vi "Impedance_Static_Temp.vi"() -> ()   [LabVIEW 2018]
uses:
  <vilib>/Utility/file.llb/Write Delimited Spreadsheet (DBL).vi
  <instrlib>/Agilent 4194/Agilent 4194.lvlib
panel:
  in  "Sample Thickness (micron)":dbl
  in  "Electrode Diameter (mm)":dbl
  out "error out":errorcluster
  out "Imaginary Permittivity":T1(graph)
  out "Real Permittivity":T1(graph)
  in  "STOP A":bool
  in  "Start Impedance Collection":bool
  in  "Gain-Phase (0:Tch/Rch [dB] - Theta)":u32(ring) items=["Tch/Rch [dB] - Theta", "Tch/Rch - theta", "Tch/Rch [dB] - tau", "Tch-Rch [V]", "Tch-Rch [dBm]", "Tch-Rch [dBV]"]
  in  "Sweep Type (F:Linear)":bool
  in  "Stop/Span (10,00E-3)":dbl=15000000.0 format="%^.1e"
  in  "Start/Center (10,00E-3)":dbl=100.0 min=-40.0 max=40000000.0 format="%^.3e"
  in  "Display Mode (0:X - A&B)":u32(ring) items=["X - A&B", "A - B", "Table"]
  in  "Number Of Points (100)":i32=400 min=2 max=401
  in  "Averaging Number (8:256)":u32(ring) items=["1", "2", "4", "8", "16", "32", "64", "128", "256"]
  in  "Integration Time (0:Short)":u32(ring) items=["Short", "Medium", "Long"]
  in  "Impedance (0:| Z | - Theta )":u32(ring) items=["| Z | -Ttheta ", "R - X", "Ls-Rs", "Ls-Q", "Cs-Rs", "Cs-Q", "Cs-D", "|Y|-Theta", "G-B", "Lp-G", "Lp-Q", "Cp-G", "Cp-Q", "Cp-D", "|Z|-Ls", "|Z|-Cs", "|Z|-Lp", "|Z|-Cp", "Lp-Rp", "Cp-Rp"]
  in  "Measurement Type (0:Impedance)":u32(ring) items=["Impedance ", "Gain - Phase", "Impedance With Probe"]
  in  "File Base Name":string
  in  "VISA resource name 2":refnum<visa-resource-name>="GPIB0::17::INSTR"
  out "Capacitance":T1(graph)
  out "Dissipation":T1(graph)
  in  "Force Quit":bool
  out "Status":string
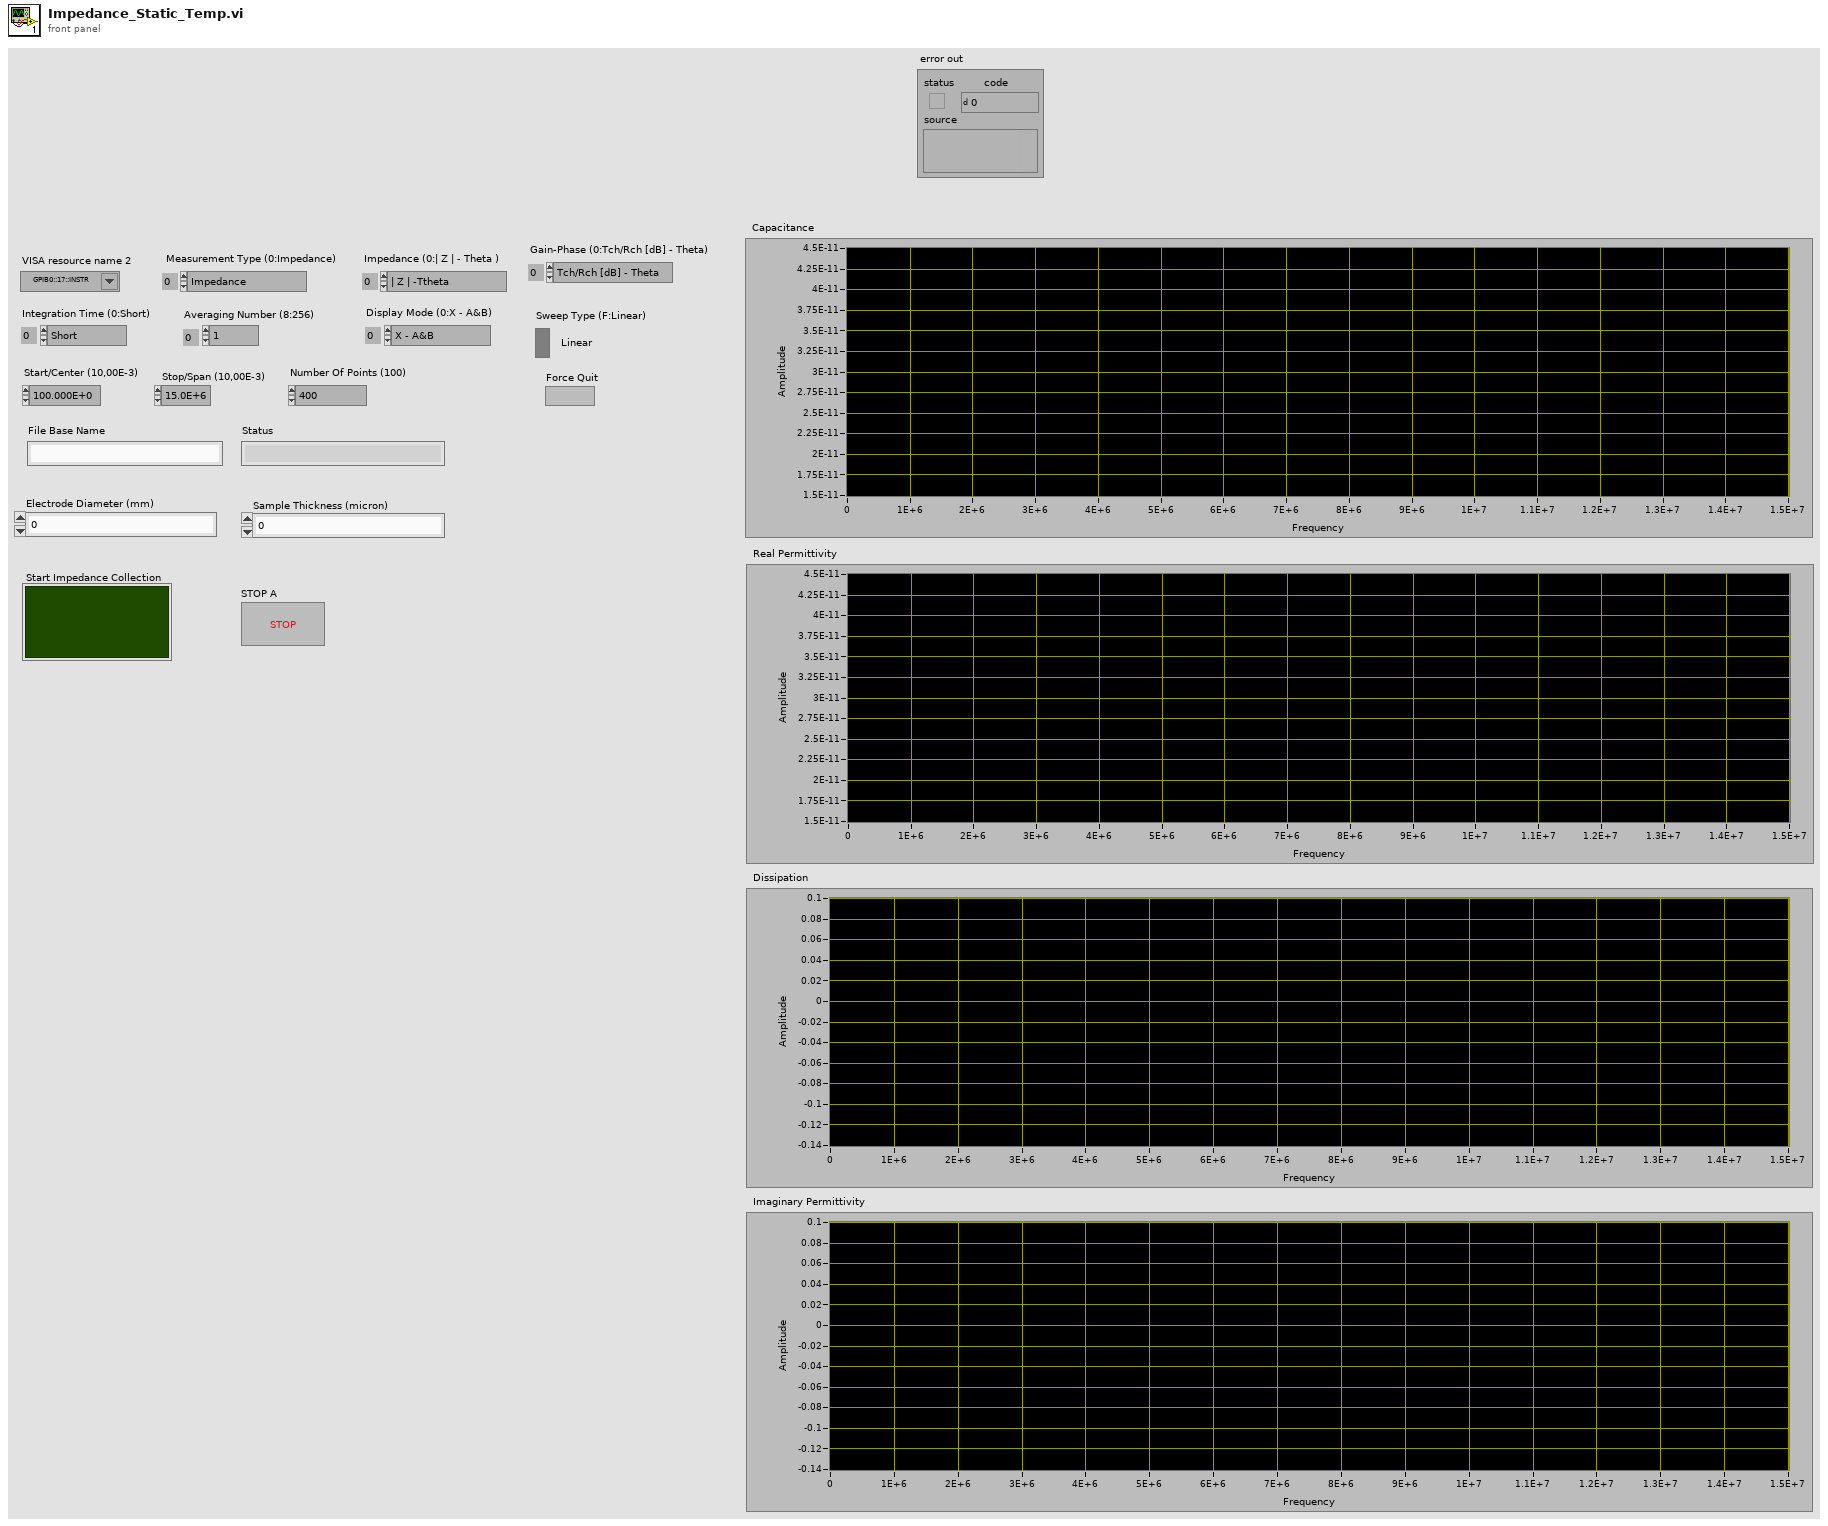
[diagram p1: front panel]
types:
  T1 = cluster{"Register Data":dbl[], "Offset/Calib Register Data":dbl[]}
  T2 = enum16{"open", "replace", "create", "open or create", "replace or create", "replace or create with confirmation"}
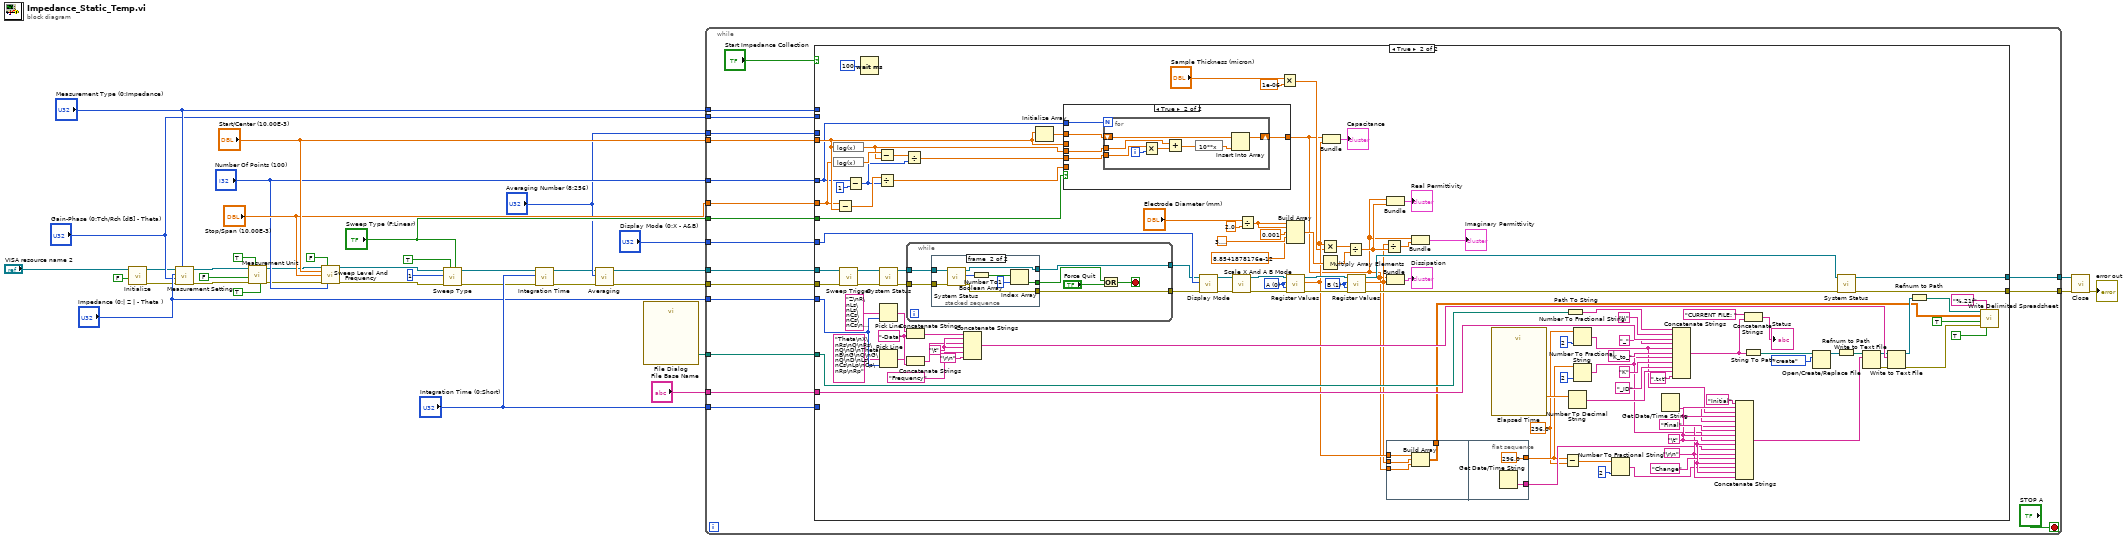
[diagram p0: block diagram]
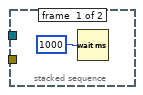
[diagram p3: hidden frame]
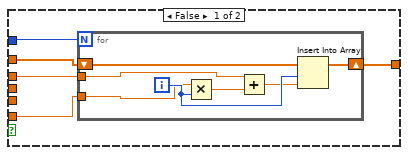
[diagram p4: hidden frame]
diagram:
  n1 = call <instrlib>:"Initialize.vi"("Reset Device (T:Reset Device)"=FALSE, "VISA resource name"="VISA resource name 2") -> ("error out"=w19:errorcluster, "VISA resource name out"=w18:refnum<visa-resource-name>)  [unwired: 8 in]
  n2 = call <instrlib>:"Measurement Setting.vi"("Measurement Type (0:Impedance)"="Measurement Type (0:Impedance)", "error in (no error)"=w19, "Gain-Phase (0:Tch/Rch [dB] - Theta)"="Gain-Phase (0:Tch/Rch [dB] - Theta)", "Impedance (0:| Z | - Theta )"="Impedance (0:| Z | - Theta )", "VISA resource name"=w18) -> ("error out"=w24:errorcluster, "VISA resource name out"=w25:refnum<visa-resource-name>)  [unwired: 5 in]
  n3 = call <instrlib>:"Measurement Unit.vi"("Test Input Impedance(T:50 ohm)"=TRUE ("Ref Attenuation (F:0 dB)"), "Power Splitter (F:Dual)"=TRUE ("Ref Attenuation (F:0 dB)"), "error in (no error)"=w24, "Ref Input Impedance (T:50 ohm)"=FALSE ("Ref Attenuation (F:0 dB)"), "VISA resource name"=w25) -> ("error out"=w22:errorcluster, "VISA resource name out"=w23:refnum<visa-resource-name>)  [unwired: 5 in]
  n4 = call <instrlib>:"Sweep Level And Frequency.vi"("VISA resource name"=w23, "Step/Number Of Points (F:Points)"=FALSE ("Step/Number Of Points (F:Points))"), "Start/Center (10,00E-3)"="Start/Center (10,00E-3)", "Stop/Span (10,00E-3)"="Stop/Span (10,00E-3)", "error in (no error)"=w22, "Number Of Points (100)"="Number Of Points (100)") -> ("VISA resource name out"=w21:refnum<visa-resource-name>, "error out"=w20:errorcluster)  [unwired: 8 in]
  n5 = call <instrlib>:"Sweep Type.vi"("Sweep Type (F:Linear)"="Sweep Type (F:Linear)", "Sweep Direction (F:Down)"=TRUE, "error in (no error)"=w20, "Sweep Mode (0:Repeat)"=u32 1, "VISA resource name"=w21) -> ("error out"=w15:errorcluster, "VISA resource name out"=w16:refnum<visa-resource-name>)  [unwired: 5 in]
  n6 = call <instrlib>:"Integration Time.vi"("error in (no error)"=w15, "Integration Time (0:Short)"="Integration Time (0:Short)", "VISA resource name"=w16) -> ("error out"=w13:errorcluster, "VISA resource name out"=w14:refnum<visa-resource-name>)  [unwired: 7 in]
  n7 = call <instrlib>:"Averaging.vi"("error in (no error)"=w13, "Averaging Number (8:256)"="Averaging Number (8:256)", "VISA resource name"=w14) -> ("error out"=w5:errorcluster, "VISA resource name out"=w4:refnum<visa-resource-name>)  [unwired: 7 in]
  n8 = call "File Dialog"() -> ("selected path"=w30:path)  [unwired: 12 in, 3 out]
  n9 = while {
    tunnel: "Start/Center (10,00E-3)" -> [w55]
    tunnel: "Stop/Span (10,00E-3)" -> [w54]
    tunnel: "Number Of Points (100)" -> [w53]
    tunnel: "Sweep Type (F:Linear)" -> [w52]
    tunnel: "Integration Time (0:Short)" -> [w51]
    tunnel: "Averaging Number (8:256)" -> [w50]
    tunnel: "Display Mode (0:X - A&B)" -> [w49]
    tunnel: w30 -> [w48]
    tunnel: "File Base Name" -> [w47]
    tunnel: "Measurement Type (0:Impedance)" -> [w46]
    tunnel: "Impedance (0:| Z | - Theta )" -> [w45]
    tunnel: "Gain-Phase (0:Tch/Rch [dB] - Theta)" -> [w44]
    tunnel: w5 -> [w41]
    tunnel: w4 -> [w40]
    tunnel: [w39] -> w2
    tunnel: [w38] -> w1
    stop <- "STOP A" stop-if-true
    n10 = case shown="True" "Start Impedance Collection" {
      tunnel: w55 -> [_ w167]
      tunnel: w54 -> [_ w166]
      tunnel: w53 -> [_ w165]
      tunnel: w52 -> [_ w164]
      tunnel: w51 -> [_ _]
      tunnel: w50 -> [_ _]
      tunnel: w49 -> [_ w163]
      tunnel: w48 -> [_ w162]
      tunnel: w47 -> [_ w161]
      tunnel: w46 -> [_ _]
      tunnel: w45 -> [_ w160]
      tunnel: w44 -> [_ _]
      tunnel: [_ w60] -> w39
      tunnel: [_ w59] -> w38
      tunnel: w41 -> [_ w58]
      tunnel: w40 -> [_ w57]
      frame False {
      }
      frame True {
        w79 = 296.0 ("In 2 Value")
        w103 = "\r\n"
        w105 = "\t"
        w135 = "-Data" ("string")
        w138 = u32 0 items=["A", "B", "C", "D", "E", "F", "G", "H", "I", "J", "RA", "RB", "RC", "RD", "RE", "RF", "RG", "RH", "RI", "RJ", "RK", "RL"] ("Registers (0:A)")
        w142 = u32 1 items=["A", "B", "C", "D", "E", "F", "G", "H", "I", "J", "RA", "RB", "RC", "RD", "RE", "RF", "RG", "RH", "RI", "RJ", "RK", "RL"] ("Registers (0:A) 2")
        w141 = "\t"
        n11 = expression code="log(x)"(w167) -> (w145:dbl)
        n12 = expression code="log(x)"(w166) -> (w148:dbl)
        n13 = Subtract(x=w166, y=w167) -> (x-y=w155:dbl)
        n14 = call <instrlib>:"Sweep Trigger.vi"("error in (no error)"=w58, "VISA resource name"=w57) -> ("error out"=w127:errorcluster, "VISA resource name out"=w128:refnum<visa-resource-name>)  [unwired: 8 in]
        n15 = Subtract(x=w165, y=1) -> (x-y=w143:i32)
        n16 = Wait (ms)(milliseconds to wait=u32 100) -> ()  [unwired: 1 out]
        n17 = Subtract(x=w148, y=w145) -> (x-y=w147:dbl)
        n18 = Divide(x=w155, y=w143) -> (x/y=w154:dbl)
        n19 = call <instrlib>:"System Status.vi"("error in (no error)"=w127, "VISA resource name"=w128) -> ("error out"=w126:errorcluster, "VISA resource name out"=w125:refnum<visa-resource-name>)  [unwired: 6 in, 2 out]
        n20 = Pick Line(multi-line string="Z\nR\nLs\nLs\nCs\nCs\nCs\nY\nG\nLp\nLp\nCp\nCp\nCp\nZ\nZ\nZ\nZ\nLp\nCp", line index=w160) -> (output string=w134:string)  [unwired: 1 in]
        n21 = Pick Line(multi-line string="Theta\nX\nRs\nQ\nRs\nQ\nD\nTheta\nB\nG\nQ\nG\nQ\nD\nLs\nCs\nLp\nCp\nRp\nRp", line index=w160) -> (output string=w133:string)  [unwired: 1 in]
        n22 = Divide(x=w147, y=w143) -> (x/y=w146:dbl)
        n23 = while {
          tunnel: w125 -> [w180]
          tunnel: w126 -> [w179]
          tunnel: [w178] -> w130
          tunnel: [w177] -> w129
          stop <- w176 stop-if-true
          n24 = stacked-sequence {
            tunnel: w180 -> [_ w189]
            tunnel: w179 -> [_ w188]
            tunnel: [_ w187] -> w178
            tunnel: [_ w186] -> w177
            tunnel: [_ w185] -> w174
            frame #0 {
              n25 = Wait (ms)(milliseconds to wait=u32 1000) -> ()  [unwired: 1 out]
            }
            frame #1 {
              n26 = call <instrlib>:"System Status.vi"("error in (no error)"=w188, "VISA resource name"=w189) -> ("error out"=w186:errorcluster, "ESR? (0)"=w184:i32, "VISA resource name out"=w187:refnum<visa-resource-name>)  [unwired: 6 in, 1 out]
              n27 = Number To Boolean Array(number=w184) -> (Boolean array=w183:bool[])
              n28 = Index Array(array=w183, index=1) -> (element=w185:bool)
            }
          }
          n29 = Or(x=w174, y="Force Quit") -> (x .or. y?=w176:bool)
        }
        n30 = Concatenate Strings(w134, w135) -> (w132:string)
        n31 = Concatenate Strings(w133, w135) -> (w131:string)
        n32 = Concatenate Strings(w132, w141, w131, w141, "Frequency" ("string"), "\r\n") -> (w112:string)
        n33 = Initialize Array(w167) -> (w156:dbl[])  [unwired: 1 in]
        n34 = case shown="True" w164 {
          tunnel: w156 -> [w194 w205]
          tunnel: w165 -> [w193 w206]
          tunnel: w154 -> [w192 _]
          tunnel: w167 -> [w191 _]
          tunnel: [w190 w204] -> w62
          tunnel: w146 -> [_ w203]
          tunnel: w145 -> [_ w202]
          frame False {
            n35 = for {
              N: w193 -> [_]
              shift-right: [w200] -> w190
              shift-left: w194 -> [w201]
              tunnel: w191 -> [w197]
              tunnel: w192 -> [w195]
              i -> [w199]
              n36 = Multiply(x=w195, y=w199) -> (x*y=w196:dbl)
              n37 = Add(x=w197, y=w196) -> (x+y=w198:dbl)
              n38 = Insert Into Array(array=w201, index=w199, new element=w198) -> (w200:dbl[])
            }
          }
          frame True {
            n39 = for {
              N: w206 -> [_]
              shift-right: [w214] -> w204
              shift-left: w205 -> [w213]
              tunnel: w203 -> [w211]
              tunnel: w202 -> [w207]
              i -> [w210]
              n40 = Multiply(x=w211, y=w210) -> (x*y=w212:dbl)
              n41 = Add(x=w207, y=w212) -> (x+y=w209:dbl)
              n42 = expression code="10**x"(w209) -> (w208:dbl)
              n43 = Insert Into Array(array=w213, new element=w208) -> (w214:dbl[])  [unwired: 1 in]
            }
          }
        }
        n44 = call <instrlib>:"Display Mode.vi"("error in (no error)"=w129, "Display Mode (0:X - A&B)"=w163, "VISA resource name"=w130) -> ("error out"=w158:errorcluster, "VISA resource name out"=w159:refnum<visa-resource-name>)  [unwired: 7 in]
        n45 = call <instrlib>:"Scale X And A B Mode.vi"("VISA resource name"=w159, "error in (no error)"=w158) -> ("VISA resource name out"=w152:refnum<visa-resource-name>, "error out"=w151:errorcluster)  [unwired: 12 in]
        n46 = Divide(x="Electrode Diameter (mm)", y=2.0) -> (x/y=w73:dbl)
        n47 = Multiply(x="Sample Thickness (micron)", y=1e-06) -> (x*y=w68:dbl)
        n48 = Build Array(w73, w73, 0.001 ("element"), 3.141592653589793, 8.8541878176e-12) -> (w76:dbl[])
        n49 = call <instrlib>:"Register Values.vi"("error in (no error)"=w151, "Calib/Offset Register (0:OFSTA)"=w138, "Registers (0:A)"=w138, "VISA resource name"=w152) -> ("error out"=w149:errorcluster, "Register Data"=w69:dbl[], "VISA resource name out"=w150:refnum<visa-resource-name>)  [unwired: 2 in, 3 out]
        n50 = Multiply(x=w69, y=w68) -> (x*y=w70:dbl[])
        n51 = Multiply Array Elements(1:w76) -> (0:w67:dbl)
        n52 = Bundle(w62, "Register Data"=w69) -> (→"Capacitance":cluster{dbl[], "Register Data":dbl[]})  [unwired: 1 in]
        n53 = Divide(x=w70, y=w67) -> (x/y=w65:dbl[])
        n54 = call <instrlib>:"Register Values.vi"("error in (no error)"=w149, "Calib/Offset Register (0:OFSTA)"=w142, "Registers (0:A)"=w142, "VISA resource name"=w150) -> ("error out"=w123:errorcluster, "Register Data"=w64:dbl[], "VISA resource name out"=w124:refnum<visa-resource-name>)  [unwired: 2 in, 3 out]
        n55 = Divide(x=w64, y=w65) -> (x/y=w63:dbl[])
        n56 = Bundle(w62, w65) -> (→"Real Permittivity":cluster{dbl[], dbl[]})  [unwired: 1 in]
        n57 = Bundle(w62, "Register Data"=w64) -> (→"Dissipation":cluster{dbl[], "Register Data":dbl[]})  [unwired: 1 in]
        n58 = flat-sequence {
          tunnel: w69 -> [w171]
          tunnel: w64 -> [w170]
          tunnel: w62 -> [w169]
          tunnel: [w168] -> w89
          tunnel: [296.0 ("In 2 Value 2")] -> w86
          tunnel: [w173] -> w88
          frame #0 {
            n59 = Build Array(w171, w170, w169) -> (w168:dbl[][])
          }
          frame #1 {
            n60 = Get Date/Time String() -> (time string=w173:string)  [unwired: 3 in, 1 out]
          }
        }
        n61 = Bundle(w62, w63) -> (→"Imaginary Permittivity":cluster{dbl[], dbl[]})  [unwired: 1 in]
        n62 = call "Elapsed Time"() -> ("Elapsed Time (s)"=w97:dbl)  [unwired: 12 in, 7 out]
        n63 = Subtract(x=w86, y=w79) -> (x-y=w83:dbl)
        n64 = Path To String(path=w162) -> (string=w122:string)
        n65 = Number To Decimal String(number=w97) -> (decimal integer string=w93:string)  [unwired: 1 in]
        n66 = Number To Fractional String(number=w79, precision (6)=i16 2) -> (F-format string=w81:string)  [unwired: 2 in]
        n67 = Number To Fractional String(number=w86, precision (6)=i16 2) -> (F-format string=w87:string)  [unwired: 2 in]
        n68 = Number To Fractional String(number=w83, precision (6)=i16 2) -> (F-format string=w84:string)  [unwired: 2 in]
        n69 = Get Date/Time String() -> (time string=w102:string)  [unwired: 3 in, 1 out]
        n70 = Concatenate Strings(w122, "\\", w161, "_", w81, "K_to_" ("string"), w87, "K" ("string"), "_ID", w93, ".txt" ("string")) -> (w90:string)
        n71 = Concatenate Strings("Initial" ("string"), w105, w81, w105, w102, w103, "Final" ("string"), w105, w87, w105, w88, w103, "Change" ("string"), w105, w84, w105, w103) -> (w99:string)
        n72 = Concatenate Strings("CURRENT FILE: " ("string"), w90) -> (→"Status":string)
        n73 = String To Path(string=w90) -> (path=w120:path)
        n74 = Open/Create/Replace File(file path (use dialog)=w120, operation (0:open)=T2."create") -> (refnum out=w101:refnum<file>)  [unwired: 4 in, 2 out]
        n75 = call <instrlib>:"System Status.vi"("error in (no error)"=w123, "VISA resource name"=w124) -> ("error out"=w60:errorcluster, "VISA resource name out"=w59:refnum<visa-resource-name>)  [unwired: 6 in, 2 out]
        n76 = Refnum to Path(1:w101) -> (0:w100:path)
        n77 = Write to Text File(file (use dialog)=w100, text=w99) -> (refnum out=w91:refnum<file>, error out=w98:errorcluster)  [unwired: 2 in, 1 out]
        n78 = Write to Text File(file (use dialog)=w91, text=w112, error in=w98) -> (refnum out=w115:refnum<file>, error out=w114:errorcluster)  [unwired: 1 in, 1 out]
        n79 = Refnum to Path(1:w115) -> (0:w116:path)
        n80 = call-poly <vilib>:"Write Delimited Spreadsheet.vi"("file path (dialog if empty)"=w116, "format (%.3f)"="%.21f", "2D data"=w89, "append to file? (new file:F)"=TRUE ("append to file? (F)"), "error in (no error)"=w114, "transpose? (no:F)"=TRUE ("transpose? (F)")) -> ()  [unwired: 8 in, 2 out]
      }
    }
  }
  n81 = call <instrlib>:"Close.vi"("error in (no error)"=w2, "VISA resource name"=w1) -> ("error out"=→"error out":errorcluster)  [unwired: 9 in]
